vi "fibonacci_series.vi"() -> ()   [LabVIEW 2019]
panel:
  out "fibonacci series":i32
  in  "Numeric":i32
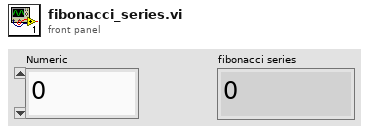
[diagram p1: front panel]
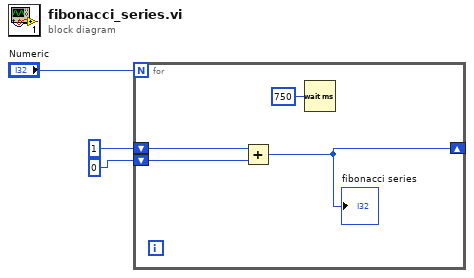
[diagram p0: block diagram]
diagram:
  n1 = for {
    N: "Numeric" -> [_]
    shift-right: [w4] -> _
    shift-left: 1 -> [w7]
    shift-left: 0 -> [w6]
    n2 = Add(x=w7, y=w6) -> (x+y=w4:i32)
    "fibonacci series" <- w4
    n3 = Wait (ms)(milliseconds to wait=u32 750) -> ()  [unwired: 1 out]
  }
